vi "test 2.vi"() -> ()   [LabVIEW 2025]
panel:
  out "VISA resource name out":refnum<visa-resource-name>
  in  "Message Based Settings:Send End Enable":bool=TRUE
  in  "Message Based Settings:Termination Character Enable":bool=TRUE
  in  "Message Based Settings:Termination Character":u8=10 format="%.0x"
  in  "Serial Settings:Flow Control":u16(ring) items=["None", "XON/XOFF", "RTS/CTS", "XON/XOFF & RTS/CTS", "DTR/DSR", "XON/XOFF & DTR/DSR"]
  in  "Serial Settings:Stop Bits":u16(ring)=10 items=["1.0"=10, "1.5"=15, "2.0"=20]
  in  "Serial Settings:Parity":u16(ring) items=["None", "Odd", "Even", "Mark", "Space"]
  in  "write buffer":string="L\\r"
  out "read buffer":string
  in  "VISA resource name":refnum<visa-resource-name>
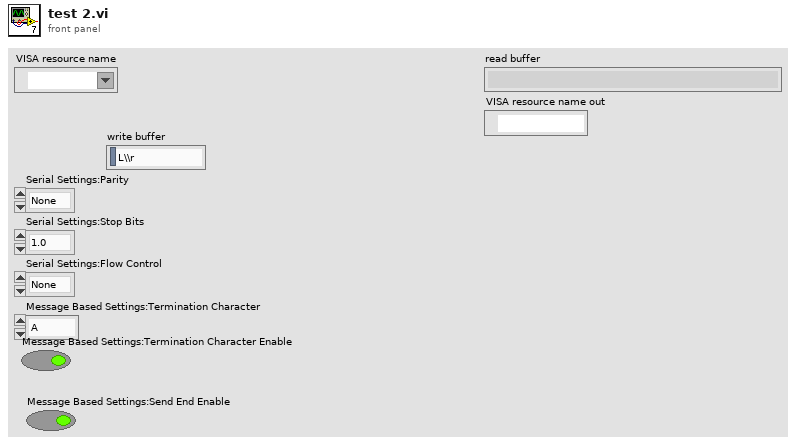
[diagram p1: front panel]
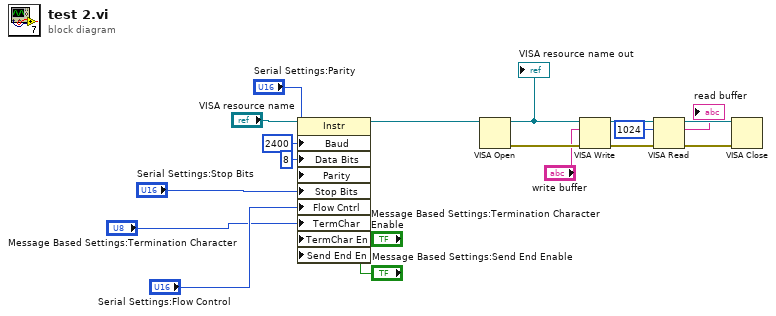
[diagram p0: block diagram]
diagram:
  n1 = property class="Instr"(reference="VISA resource name", "Baud"=u32 2400 ("Serial Settings:Baud Rate"), "Data Bits"=u16 8 ("Serial Settings:Data Bits"), "Parity"="Serial Settings:Parity", "Stop Bits"="Serial Settings:Stop Bits", "Flow Cntrl"="Serial Settings:Flow Control", "TermChar"="Message Based Settings:Termination Character", "TermChar En"="Message Based Settings:Termination Character Enable", "Send End En"="Message Based Settings:Send End Enable") -> (reference out=w11:refnum<visa-resource-name>)  [unwired: 1 in, 1 out]
  n2 = VISA Open(VISA resource name=w11) -> (VISA resource name=w10:refnum<visa-resource-name>, error out=w9:errorcluster)  [unwired: 4 in]
  "VISA resource name out" <- w10
  n3 = VISA Write(VISA resource name=w10, write buffer="write buffer", error in (no error)=w9) -> (VISA resource name out=w7:refnum<visa-resource-name>, error out=w6:errorcluster)  [unwired: 1 out]
  n4 = VISA Read(VISA resource name=w7, byte count=u32 1024, error in (no error)=w6) -> (VISA resource name out=w4:refnum<visa-resource-name>, read buffer=→"read buffer":string, error out=w5:errorcluster)  [unwired: 1 out]
  n5 = VISA Close(VISA resource name=w4, error in (no error)=w5) -> ()  [unwired: 1 out]
